vi "Place dots fixed.vi"(6 "Right Corner":cluster{"X":sgl, "Y":sgl}[](array[cluster]), 8 "Left Height":dbl, 9 "Left Orientation":dbl, 10 "Left Corner":cluster{"X":sgl, "Y":sgl}[](array[cluster]), 11 "Image IN":T1) -> (3 "Image OUT":T1)   [LabVIEW 2018]
uses:
  <vilib>/vision/Image Controls.llb/IMAQ Image.ctl
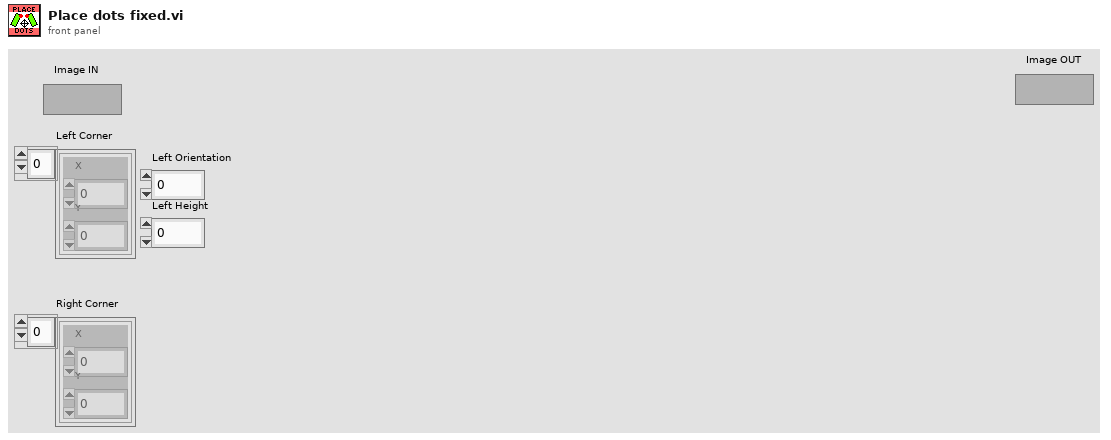
[diagram p1: front panel]
types:
  T1 = typedef "IMAQ Image.ctl" = refnum<image>
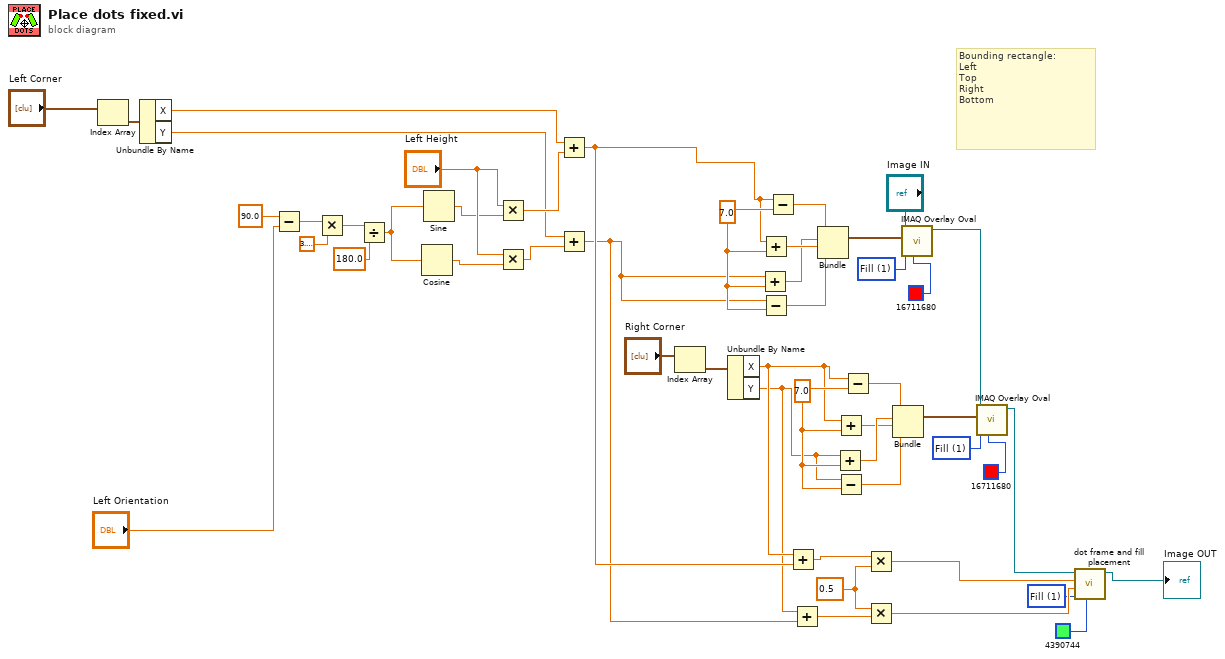
[diagram p0: block diagram]
diagram:
  w1 = u32 1 items=["Frame", "Fill"] ("Drawing Mode (Frame)")
  w8 = 0.5 ("x")
  w31 = u32 1 items=["Frame", "Fill"] ("Drawing Mode (Frame)")
  w35 = sgl 7.0 ("y")
  w47 = u32 1 items=["Frame", "Fill"] ("Drawing Mode (Frame)")
  w43 = sgl 7.0 ("y")
  # "Bounding rectangle:\nLeft\nTop\nRight\nBottom"
  n1 = Index Array(array="Left Corner") -> (element=w40:cluster{"X":sgl, "Y":sgl})  [unwired: 1 in]
  n2 = Unbundle By Name(w40) -> ("X"=w16:sgl, "Y"=w15:sgl)
  n3 = Subtract(x=90.0, y="Left Orientation") -> (x-y=w26:dbl)
  n4 = Multiply(x=w26, y=3.141592653589793) -> (x*y=w24:dbl)
  n5 = Divide(x=w24, y=180.0) -> (x/y=w22:dbl)
  n6 = Cosine(x=w22) -> (cos(x)=w19:dbl)
  n7 = Sine(x=w22) -> (sin(x)=w20:dbl)
  n8 = Multiply(x="Left Height", y=w20) -> (x*y=w18:dbl)
  n9 = Multiply(x="Left Height", y=w19) -> (x*y=w17:dbl)
  n10 = Add(x=w16, y=w18) -> (x+y=w13:dbl)
  n11 = Add(x=w15, y=w17) -> (x+y=w11:dbl)
  n12 = Index Array(array="Right Corner") -> (element=w37:cluster{"X":sgl, "Y":sgl})  [unwired: 1 in]
  n13 = Unbundle By Name(w37) -> ("X"=w12:sgl, "Y"=w10:sgl)
  n14 = Add(x=w11, y=w43) -> (x+y=w44:dbl)
  n15 = Add(x=w13, y=w43) -> (x+y=w45:dbl)
  n16 = Subtract(x=w11, y=w43) -> (x-y=w42:dbl)
  n17 = Subtract(x=w13, y=w43) -> (x-y=w46:dbl)
  n18 = Add(x=w12, y=w13) -> (x+y=w9:dbl)
  n19 = Add(x=w10, y=w11) -> (x+y=w2:dbl)
  n20 = Bundle(w46, w44, w45, w42) -> (w48:cluster{dbl, dbl, dbl, dbl})  [unwired: 1 in]
  n21 = Add(x=w10, y=w35) -> (x+y=w34:sgl)
  n22 = Add(x=w12, y=w35) -> (x+y=w33:sgl)
  n23 = Subtract(x=w10, y=w35) -> (x-y=w36:sgl)
  n24 = Subtract(x=w12, y=w35) -> (x-y=w32:sgl)
  n25 = Multiply(x=w9, y=w8) -> (x*y=w5:dbl)
  n26 = Multiply(x=w8, y=w2) -> (x*y=w4:dbl)
  n27 = Bundle(w32, w34, w33, w36) -> (w30:cluster{sgl, sgl, sgl, sgl})  [unwired: 1 in]
  n28 = call "IMAQ Overlay Oval"("Color"=u32 16711680 ("Side colors"), "Drawing Mode (Frame)"=w47, "Bounding Rectangle"=w48, "Image"="Image IN") -> ("Image Out"=w28:T1)  [unwired: 6 in, 1 out]
  n29 = call "IMAQ Overlay Oval"("Color"=u32 16711680 ("Side colors"), "Drawing Mode (Frame)"=w31, "Bounding Rectangle"=w30, "Image"=w28) -> ("Image Out"=w7:T1)  [unwired: 6 in, 1 out]
  n30 = call "dot frame and fill placement.vi"("Color"=u32 4390744, "Drawing Mode (Frame)"=w1, "y coordinate"=w4, "x coordinate"=w5, "Image"=w7) -> ("Image Out"=→"Image OUT":T1)  [unwired: 6 in]
